vi "打开串口错误.vi"(10 "消息数据":variant, 11 "队列输入":refnum<queue>) -> ()   [LabVIEW 2016]
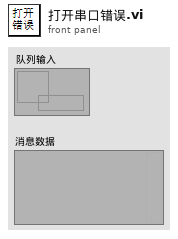
[diagram p1: front panel]
types:
  T1 = typedef "串口事件状态控件.ctl" = cluster{"串口状态":enum16{"打开串口", "关闭串口", "串口接收", "打开错误"}, "消息数据":variant}
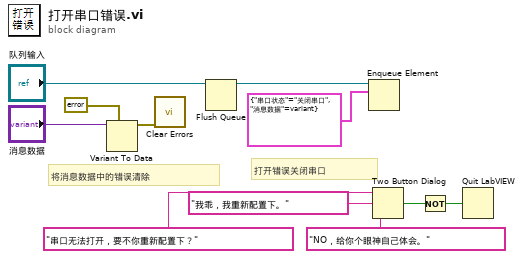
[diagram p0: block diagram]
diagram:
  # "打开错误关闭串口"
  # "将消息数据中的错误清除"
  n1 = Variant To Data(type=errorcluster {"status"=FALSE, "code"=0, "source"=""} ("错误输入"), Variant="消息数据") -> (data=w5:errorcluster)  [unwired: 1 in, 1 out]
  n2 = call <vilib>:"Clear Errors.vi"("error in (no error)"=w5) -> ()  [unwired: 5 in, 2 out]
  n3 = Flush Queue(queue="队列输入") -> (queue out=w2:refnum<queue>)  [unwired: 1 in, 2 out]
  n4 = Enqueue Element(queue=w2, element=T1 {"串口状态"=enum."关闭串口", "消息数据"=variant}) -> ()  [unwired: 2 in, 3 out]
  n5 = Two Button Dialog(message="串口无法打开，要不你重新配置下？" ("消息"), 1:"NO，给你个眼神自己体会。" ("F按钮名称（“取消”）"), 2:"我乖，我重新配置下。" ("T按钮名称（“确定”）")) -> (T button?=w10:bool)
  n6 = Not(x=w10) -> (.not. x?=w11:bool)
  n7 = Quit LabVIEW(quit? (T)=w11) -> ()
